vi "SetParam.vi"(8 "error in (no error)":errorcluster caption="entrée d'erreur (pas d'erreur)", 10 "FunctionTransformer":T1={"func_callable"="None", "inverse_func_callable"="None", "validate"=FALSE, "accept_sparse"=FALSE, "check_inverse"=TRUE, "kw_args"={"key"=[], "Value"=[]}, "inv_kw_args"={"key"=[], "Value"=[]}}, 11 "FunctionTransformer.lvclass":refnum<class "FunctionTransformer.lvclass">) -> (0 "error in (no error)":errorcluster caption="entrée d'erreur (pas d'erreur)", 3 "FunctionTransformer.lvclass":refnum<class "FunctionTransformer.lvclass">)   [LabVIEW 2020, in "FunctionTransformer.lvclass"]
doc: "Set parameters"
uses:
  FunctionTransformer.lvclass
  FunctionTransformer.lvclass/FunctionTransformer.ctl
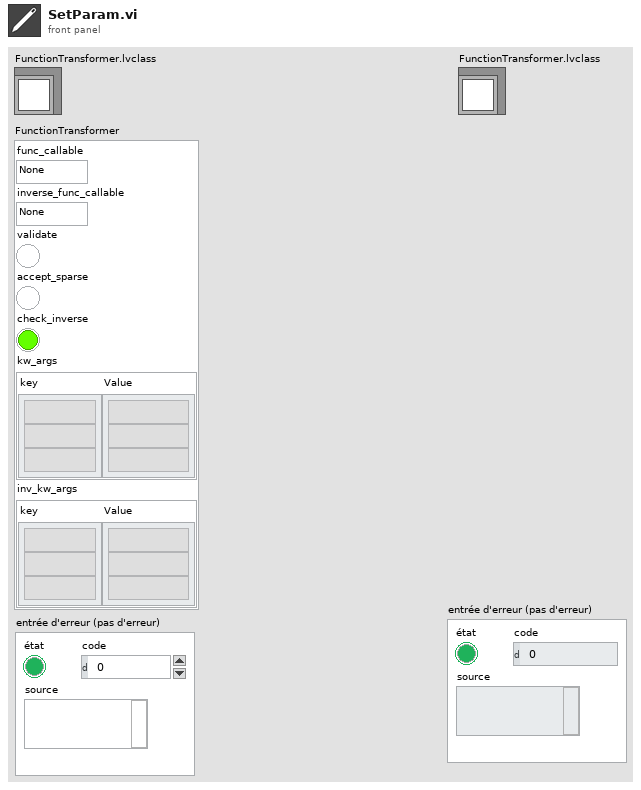
[diagram p1: front panel]
types:
  T1 = cluster{"func_callable":string, "inverse_func_callable":string, "validate":bool, "accept_sparse":bool, "check_inverse":bool, "kw_args":cluster{"key":string[], "Value":string[]}, "inv_kw_args":cluster{"key":string[], "Value":string[]}}
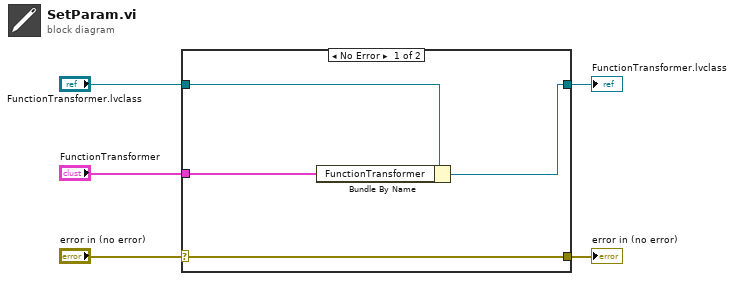
[diagram p0: block diagram]
diagram:
  n1 = case shown="No Error" "error in (no error)" {
    selector: "error in (no error)" -> [w9 w10]
    tunnel: [w9 w10] -> w4
    tunnel: [w7 w11] -> w2
    tunnel: "FunctionTransformer.lvclass" -> [w8 w11]
    tunnel: "FunctionTransformer" -> [w6 _]
    frame No Error {
      n2 = Bundle By Name(cluster=w8, "FunctionTransformer"=w6) -> (w7:refnum<class "FunctionTransformer.lvclass">)
    }
    frame Error {
    }
  }
  "error in (no error)" <- w4
  "FunctionTransformer.lvclass" <- w2
